vi "Avocent_send_cmd.vi"(8 "error in":errorcluster, 9 "timeout ms":i32=6000, 10 "Avocent IP (in)":string, 11 "HTTP command":string) -> (0 "error out":errorcluster, 2 "Avocent IP (out)":string, 3 "Replay":string)   [LabVIEW 2020]
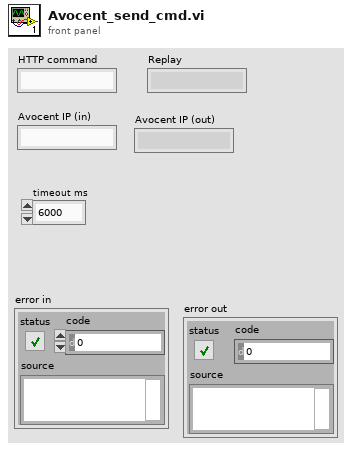
[diagram p1: front panel]
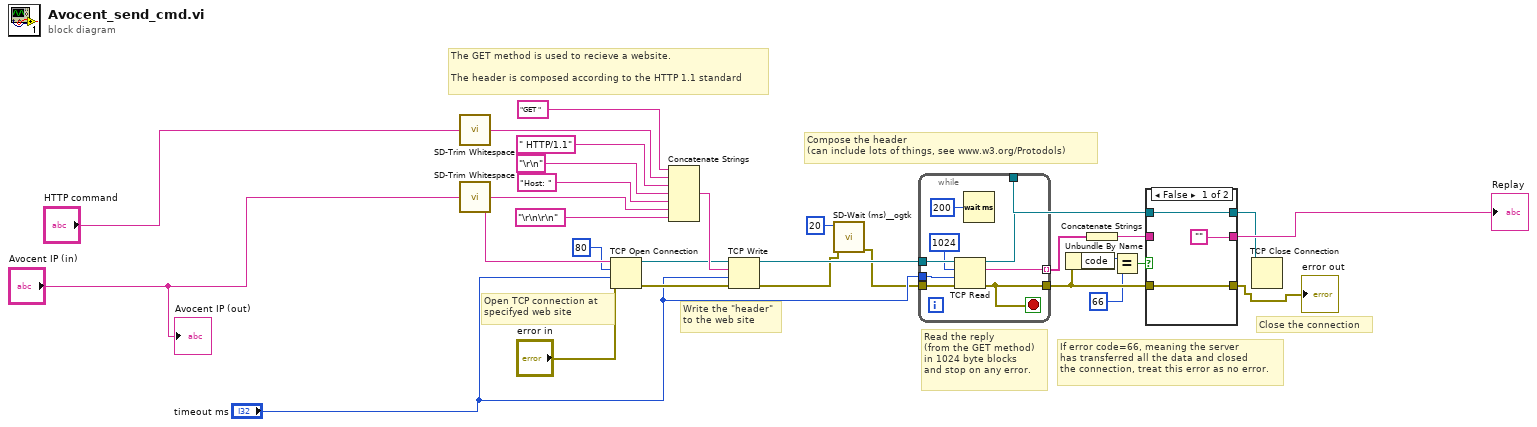
[diagram p0: block diagram]
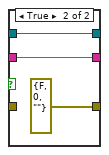
[diagram p2: hidden frame]
diagram:
  # "Compose the header\n(can include lots of things, see www.w3.org/Protodols)"
  # "The GET method is used to recieve a website.\n\nThe header is composed according to the HTTP 1.1 standard"
  # "Close the connection"
  # "If error code=66, meaning the server\nhas transferred all the data and closed\nthe connection, treat this error as no error."
  # "Read the reply\n(from the GET method)\nin 1024 byte blocks\nand stop on any error."
  # "Write the \"header\"\nto the web site"
  # "Open TCP connection at\nspecifyed web site"
  n1 = call "SD-Trim Whitespace.vi"("string"="HTTP command") -> ("trimmed string"=w27:string)  [unwired: 1 in]
  n2 = call "SD-Trim Whitespace.vi"("string"="Avocent IP (in)") -> ("trimmed string"=w28:string)  [unwired: 1 in]
  n3 = TCP Open Connection(address=w28, remote port or service name=u16 80 ("remote port"), timeout ms (60000)="timeout ms", error in (no error)="error in") -> (connection ID=w9:refnum<k5>, error out=w8:errorcluster)  [unwired: 1 in]
  n4 = Concatenate Strings("GET " ("Command"), w27, " HTTP/1.1" ("Command"), "\r\n" ("string"), "Host: " ("Command"), w28, "\r\n\r\n" ("string")) -> (w25:string)
  n5 = TCP Write(connection ID=w9, data in=w25, error in (no error)=w8, 9:"timeout ms") -> (connection ID out=w12:refnum<k5>, error out=w4:errorcluster)  [unwired: 1 out]
  n6 = call "SD-Wait (ms)__ogtk.vi"("error in (no error)"=w4, "milliseconds to wait"=u32 20) -> ("error out"=w3:errorcluster)  [unwired: 8 in, 1 out]
  n7 = while {
    tunnel: w3 -> [w37]
    tunnel: w12 -> [w36]
    tunnel: [w33] -> w14
    tunnel: [w35] -> w17
    tunnel: [w34] -> w15 mode=indexing
    tunnel: "timeout ms" -> [w32]
    stop <- w33 stop-if-true
    n8 = TCP Read(connection ID=w36, bytes to read=1024, error in (no error)=w37, 9:w32) -> (connection ID out=w35:refnum<k5>, data out=w34:string, error out=w33:errorcluster)  [unwired: 1 in]
    n9 = Wait (ms)(milliseconds to wait=u32 200) -> ()  [unwired: 1 out]
  }
  n10 = Unbundle By Name(w14) -> ("code"=w10:i32)
  n11 = Concatenate Strings(w15) -> (w16:string)
  n12 = Equal?(x=w10, y=66) -> (x = y?=w11:bool)
  n13 = case shown="False" w11 {
    tunnel: ["" w42] -> w20
    tunnel: w16 -> [_ w42]
    tunnel: [w39 errorcluster {"status"=FALSE, "code"=0, "source"=""} ("error in (no error)")] -> w1
    tunnel: w14 -> [w39 _]
    tunnel: w17 -> [w38 w41]
    tunnel: [w38 w41] -> w18
    frame False {
    }
    frame True {
    }
  }
  "Replay" <- w20
  "error out" <- w1
  n14 = TCP Close Connection(connection ID=w18) -> ()  [unwired: 2 in, 2 out]
  "Avocent IP (out)" <- "Avocent IP (in)"
